vi "picoOpen.vi"(8 "error in (no error)":errorcluster) -> (0 "error out":errorcluster, 1 "Unit Info":T1, 2 "maxADC":i16, 3 "Handle Out":i16)   [LabVIEW 2011]
uses:
  PS2000a.dll
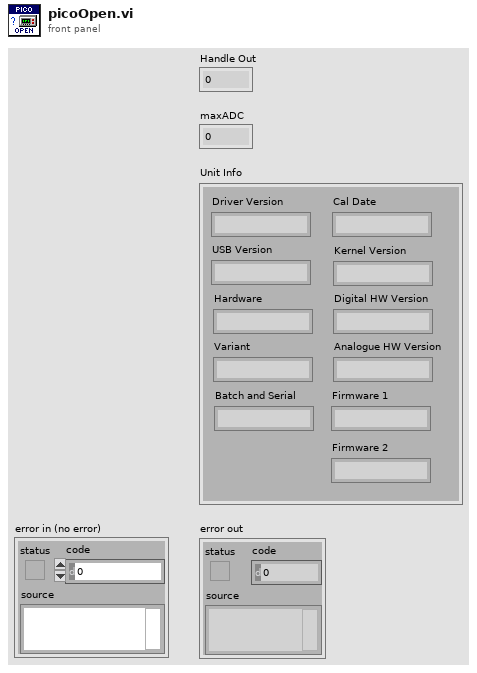
[diagram p1: front panel]
types:
  T1 = cluster{"Driver Version":string, "USB Version":string, "Hardware":string, "Variant":string, "Batch and Serial":string, "Cal Date":string, "Kernel Version":string, "Digital HW Version":string, "Analogue HW Version":string, "Firmware 1":string, "Firmware 2":string}
  T2 = cluster{"[0]":string, "[1]":string, "[2]":string, "[3]":string, "[4]":string, "[5]":string, "[6]":string, "[7]":string, "[8]":string, "[9]":string, "[10]":string}
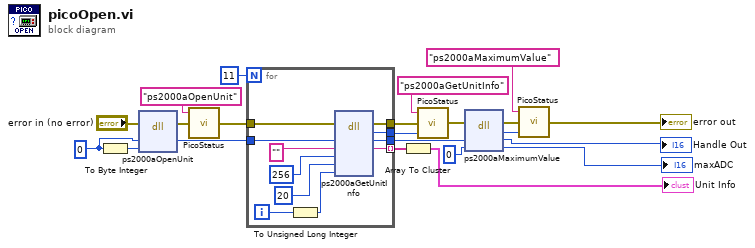
[diagram p0: block diagram]
diagram:
  w6 = i16 0 ("handle")
  n1 = To Byte Integer(number=w6) -> (8bit integer=w4:i8)
  n2 = dll-call lib="ps2000a.dll" fn="ps2000aOpenUnit" ("ps3000.dll:_ps3000_open_unit@0")(error in="error in (no error)", "handle"=w6, "serial"=w4) -> (error out=w8:errorcluster, "handle"=w5:i16)  [unwired: 4 in, 1 out]
  n3 = call "PicoStatus.vi"("error in"=w8, "source"="ps2000aOpenUnit") -> ("error out"=w9:errorcluster)  [unwired: 1 in]
  n4 = for {
    N: 11 ("PICO_INFO: 0 -10") -> [_]
    tunnel: w5 -> [w33]
    tunnel: [w30] -> w2 mode=indexing
    tunnel: w9 -> [w27]
    tunnel: [w26] -> w14
    tunnel: [w25] -> w10
    tunnel: [w24] -> w11
    i -> [w28]
    n5 = To Unsigned Long Integer(number=w28) -> (unsigned 32bit integer=w23:u32)
    n6 = dll-call lib="PS2000a.dll" fn="ps2000aGetUnitInfo"(error in=w27, "handle"=w33, "unitInfo"="", "stringLength"=i16 256, "requiredSize"=i16 20 ("stringLength"), "PICO_INFO"=w23) -> (error out=w25:errorcluster, "PICO_STATUS"=w24:u32, "handle"=w26:i16, "unitInfo"=w30:string)  [unwired: 5 in, 1 out]
  }
  n7 = Array To Cluster(array=w2) -> (cluster=→"Unit Info":T2)
  n8 = call "PicoStatus.vi"("PICO STATUS"=w11, "error in"=w10, "source"="ps2000aGetUnitInfo") -> ("error out"=w13:errorcluster)
  n9 = dll-call lib="ps2000a.dll" fn="ps2000aMaximumValue"(error in=w13, "handle"=w14, "value"=i16 0) -> (error out=w15:errorcluster, "PICO_STATUS"=w17:u32, "handle"=→"Handle Out":i16, "value"=→"maxADC":i16)  [unwired: 2 in, 1 out]
  n10 = call "PicoStatus.vi"("PICO STATUS"=w17, "error in"=w15, "source"="ps2000aMaximumValue") -> ("error out"=→"error out":errorcluster)
